vi "Enable_Visible Buttons.vi"(5 "Visible? (T)":bool=TRUE, 7 "Enable? (T)":bool=TRUE, 11 "Controls Ref Array":refnum<vi>[](array[refnum])) -> ()   [LabVIEW 2019]
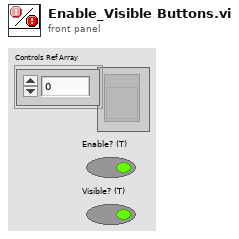
[diagram p1: front panel]
types:
  T1 = enum8{"Enabled", "Disabled", "Disabled and Grayed Out"}
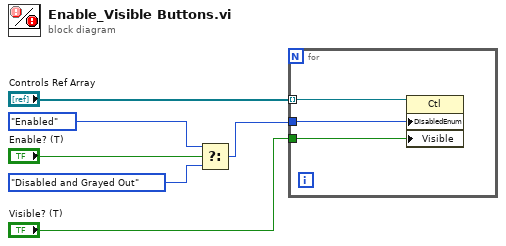
[diagram p0: block diagram]
diagram:
  n1 = Select(t=T1."Enabled" ("Disabled"), s="Enable? (T)", f=T1."Disabled and Grayed Out" ("Disabled")) -> (s? t:f=w5:T1)
  n2 = for {
    tunnel: "Controls Ref Array" -> [w9] mode=indexing
    tunnel: w5 -> [w8]
    tunnel: "Visible? (T)" -> [w7]
    n3 = property class="Ctl"(reference=w9, "DisabledEnum"=w8, "Visible"=w7) -> ()  [unwired: 1 in, 2 out]
  }
